vi "BeamBlockers.vi"() -> ()   [LabVIEW 2017]
panel:
  in  "Array":dbl[](array[numeric])
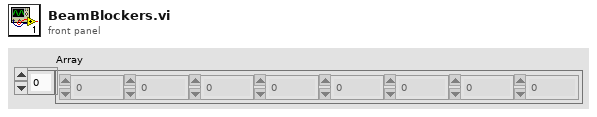
[diagram p1: front panel]
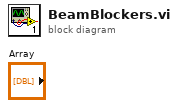
[diagram p0: block diagram]
diagram:
